vi "meta range push back.vi"(8 "error in (no error)":errorcluster, 10 "range":cluster{"start":dbl, "stop":dbl, "step":dbl}, 11 "h":u64) -> (0 "error out":errorcluster, 3 "function return":u32(ring))   [LabVIEW 2023, in "uhd.lvlib"]
doc: "UHD_API uhd_error uhd_meta_range_push_back(\n uhd_meta_range_handle h, const uhd_range_t* range);"
uses:
  <userlib>/uhd/uhd.lvlib
  <userlib>/uhd/uhd.dll
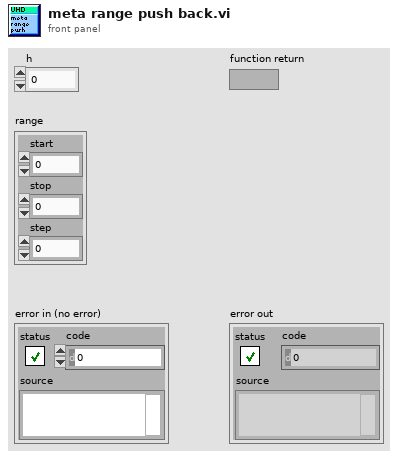
[diagram p1: front panel]
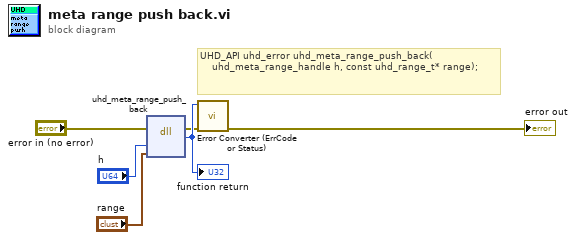
[diagram p0: block diagram]
diagram:
  # "UHD_API uhd_error uhd_meta_range_push_back(\n    uhd_meta_range_handle h, const uhd_range_t* range);"
  n1 = dll-call lib="C:/Program Files/National Instruments/LabVIEW 2023/user.lib/uhd/uhd.*" fn="uhd_meta_range_push_back"(error in="error in (no error)", "h"="h", "range"="range") -> (error out=w2:errorcluster, w6:u32)  [unwired: 4 in, 1 out]
  "function return" <- w6
  n2 = call <userlib>:"Error Converter (ErrCode or Status).vi"("error in (no error)"=w2, "error code"=w6) -> ("error out"=→"error out":errorcluster)  [unwired: 9 in]
